vi "Husky Loop.vi"() -> ()   [LabVIEW 2012]
uses:
  clearpath_interface.lvlib
  <vilib>/Platform/TimedLoop/XDataNode/XDataNode.xnode
  <vilib>/Platform/TimedLoop/XDataNode/nitl_modes.ctl
  <vilib>/Platform/TimedLoop/XDataNode/XDNodeRunTimeDep.lvlib
  <vilib>/Platform/TimedLoop/XDataNode/wakeup.ctl
  <vilib>/Platform/TimedLoop/XDataNode/timing_clust.ctl
panel:
  out "Flags":u8 format="%b"
  out "Capacity":i16
  out "Charge":dbl(slide) scale=0.0..100.0
  in  "Debug":bool
  in  "VISA resource name":refnum<visa-resource-name>
  out "Telemetry":T1={"Voltage"={0.0, 0.0, 0.0}, "Encoder Speed"={0, 0}, "Temps"={"IC Temp (C)"=0, "Ch1 Temp (C)"=0, "Ch2 Temp (C)"=0}, "Current"={0.0, 0.0, 0.0, 4.6238981750249924e+36}} {"Current" scale=0.0..16.0; "Temps"."IC Temp (C)" scale=0.0..150.0; "Temps"."Ch1 Temp (C)" scale=0.0..150.0; "Temps"."Ch2 Temp (C)" scale=0.0..150.0; "Encoder Speed" scale=-100.0..100.0; "Voltage" scale=8.0..14.0}
  in  "End Loop":bool
  in  "stop?":bool
  in  "Reset":bool
  in  "Max Accel":dbl
  in  "Set Max Accel":bool
  in  "Max Speed":dbl
  in  "Set Max Speed":bool
  in  "Set Velocity":bool
  in  "Translational Speed":dbl
  in  "Rotational Speed":dbl
  in  "Set Brake":bool
  in  "Continuous Vel":bool
  in  "Right Output":dbl
  in  "Left Output":dbl
  in  "Continuous Output":bool
  in  "Set Output":bool
  in  "P":dbl
  in  "I":dbl
  in  "D":dbl
  in  "FF":dbl
  in  "Stic":dbl
  in  "Int Lim":dbl
  in  "Set Controls":bool
  in  "Right Speed":dbl
  in  "Left Speed":dbl
  in  "Left Accel":dbl
  in  "Right Accel":dbl
  in  "Continuous Speeds":bool
  in  "Set Speeds":bool
  in  "Remote E-Stop":bool
  in  "Set Safety":bool
  in  "New Chassis Time (ms)":u32
  in  "Set Time":bool
  in  "New Chassis Name":string
  in  "Set Name":bool
  in  "FreqRawEncoder":u8
  in  "Update Raw Encoders":bool
  in  "Update Encoder":bool
  in  "FreqEncoder":u8
  in  "FreqPlatformRot":u8
  in  "Update Platform Rotation":bool
  in  "FreqMaxAccel":u8
  in  "Update Max Accel":bool
  in  "FreqMaxSpeed":u8
  in  "Update Max Speed":bool
  in  "FreqDifferentialOutput":u8
  in  "Update Differential Output":bool
  in  "FreqDifferentialControl":u8
  in  "Update Differential Control":bool
  in  "FreqDifferentialSpeed":u8
  in  "Update Differential Speed":bool
  in  "FreqSafetyStatus":u8
  in  "Update Safety Status":bool
  in  "FreqPowerSystem":u8
  in  "Update Power System":bool
  in  "FreqSystemStatus":u8
  in  "Update System Status":bool
  in  "FreqFirmwareInfo":u8
  in  "Update Firmware Info":bool
  in  "FreqPlatformName":u8
  in  "Update Platform Name":bool
  in  "FreqPlatformInfo":u8
  in  "Update Platform Info":bool
  # "Communication Status"
  # "Set Velocity"
  # "Set Differential Speeds"
  # "Set Chassis Name/Time"
  # "Set Differential Controls"
  # "Set Differential Output"
  # "Set Max Speed/Accel"
  # "Set Safety System"
  # "Reset Processor"
  # "Control Test Panel\nClearpath Control Protocol cRIO Test Interface v1.0\nClearpath Robotics Inc., (c) 2010"
  # "Subscriptions"
  # "Platform Info (0x8001)"
  # "Differential Control (0x8201)"
  # "Platform Name (0x8002)"
  # "Differential Output (0x8202)"
  # "Firmware Info (0x8003)"
  # "Max Speed (0x8210)"
  # "System Status (0x8004)"
  # "Max Accel (0x8211)"
  # "Power System (0x8005)"
  # "Platform Rotation (0x8601)"
  # "Safety System Status (0x8010)"
  # "Encoders (0x8800)"
  # "Differential Speed (0x8200)"
  # "Raw Encoders (0x8801)"
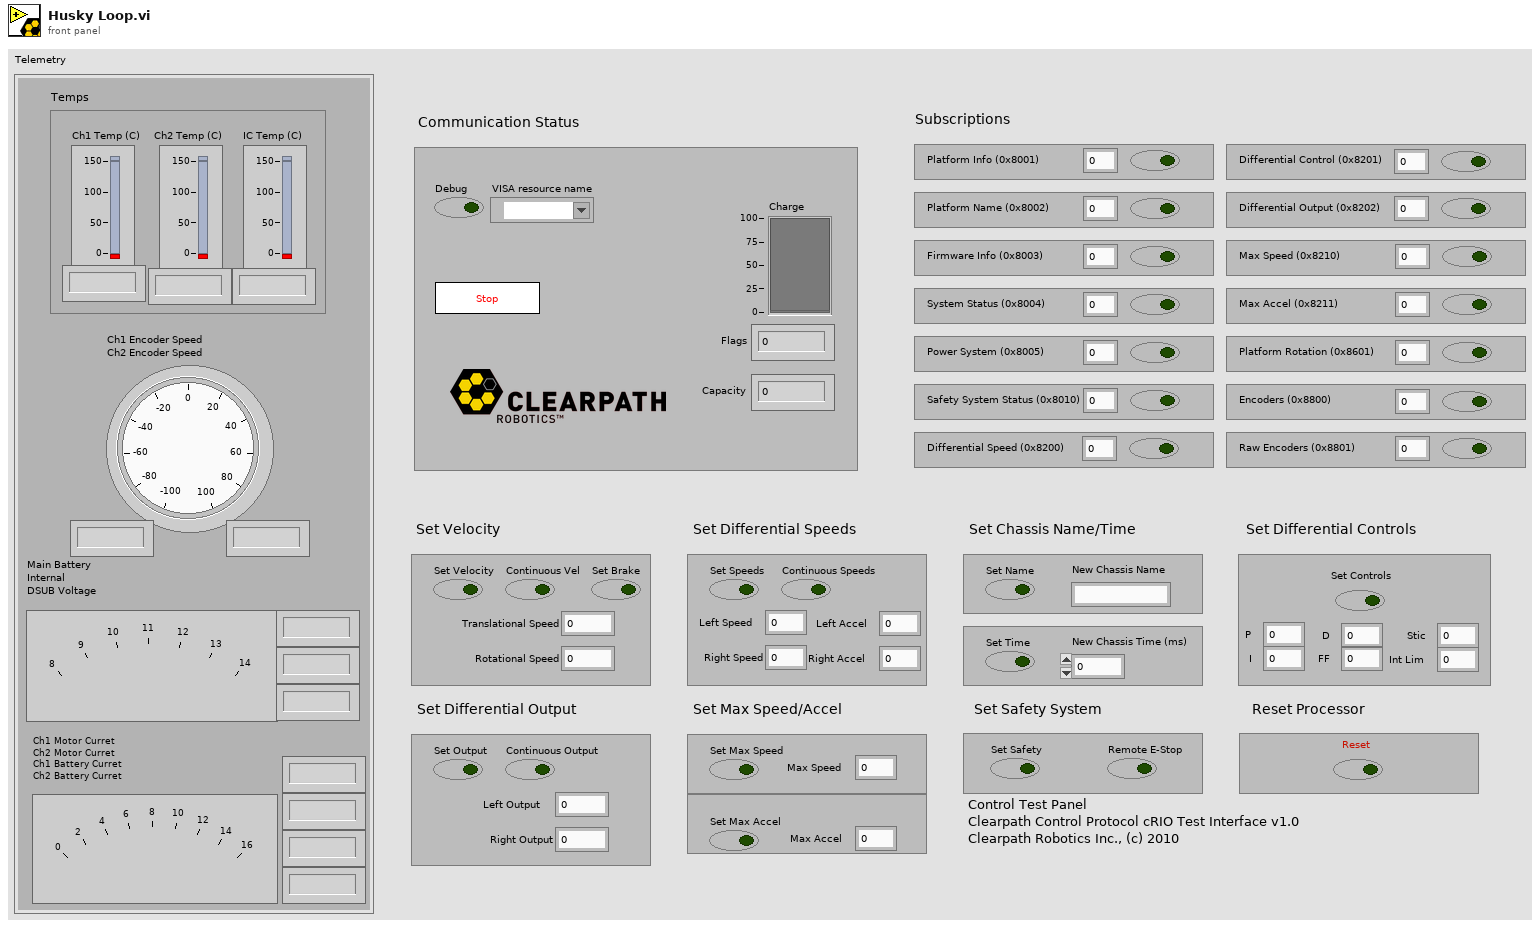
[diagram p1: front panel]
types:
  T1 = cluster{"Voltage":cluster{sgl, sgl, sgl}, "Encoder Speed":cluster{i32, i32}, "Temps":cluster{"IC Temp (C)":i32, "Ch1 Temp (C)":i32, "Ch2 Temp (C)":i32}, "Current":cluster{dbl, dbl, dbl, dbl}}
  T2 = cluster{"Xmit Queue":refnum<queue>, "Data Queue":refnum<queue>, "VISA resource name out":refnum<visa-resource-name>, "error out":errorcluster, "Message Data Cluster":cluster{"\nChar Idx":u8, "Num. Char Rem":u8, "Write Index":u8, "Read Index":u8, "Message Data Buffer":u8[][]}}
  T3 = typedef "XDNodeRunTimeDep.lvlib/timing_clust.ctl" = cluster{"Expected End [f-1]":u64, "Actual End [f-1]":u64, "Finished Late? [f-1]":bool, "Expected End [i-1]":u64, "Actual End [i-1]":u64, "Finished Late? [i-1]":bool, "Expected Start [i]":u64, "Actual Start [i]":u64, "Expected Start [f]":u64, "Actual Start [f]":u64, "Source Name":string, "Structure Name":string, "Period":i64, "Deadline":i64, "Offset":i64, "Start":i64, "Priority":i32, "Timeout":i32, "Mode":T4, "Wakeup Reason":T5, "Error":errorcluster, "Source Type":string, "Secondary Source Type":string, "Global End Time":u64, "Global Start Time":u64, "Frame Duration":u64, "Iteration Duration":u64, "Assigned CPU":i32, "I/O Scan Engine Mode":u32}
  T4 = typedef "XDNodeRunTimeDep.lvlib/nitl_modes.ctl" = enum32{"No Change", "Process missed periods, maintain original phase", "Discard missed periods, maintain original phase", "Process missed periods, ignore original phase", "Discard missed periods, ignore original phase"}
  T5 = typedef "XDNodeRunTimeDep.lvlib/wakeup.ctl" = enum32{"Normal", "Aborted", "Asynchronous wakeup", "Timing source error", "Timed loop error", "Timeout"}
  T6 = cluster{"P":dbl, "I":dbl, "D":dbl, "FF":dbl, "Stic":dbl, "Int Lim":dbl}
  T7 = cluster{"r_p":dbl, "r_i":dbl, "r_d":dbl, "r_ffwd":dbl, "r_stic":dbl, "r_int_lim":dbl}
  T8 = cluster{"l_p":dbl, "l_i":dbl, "l_d":dbl, "l_ffwd":dbl, "l_stic":dbl, "l_int_lim":dbl}
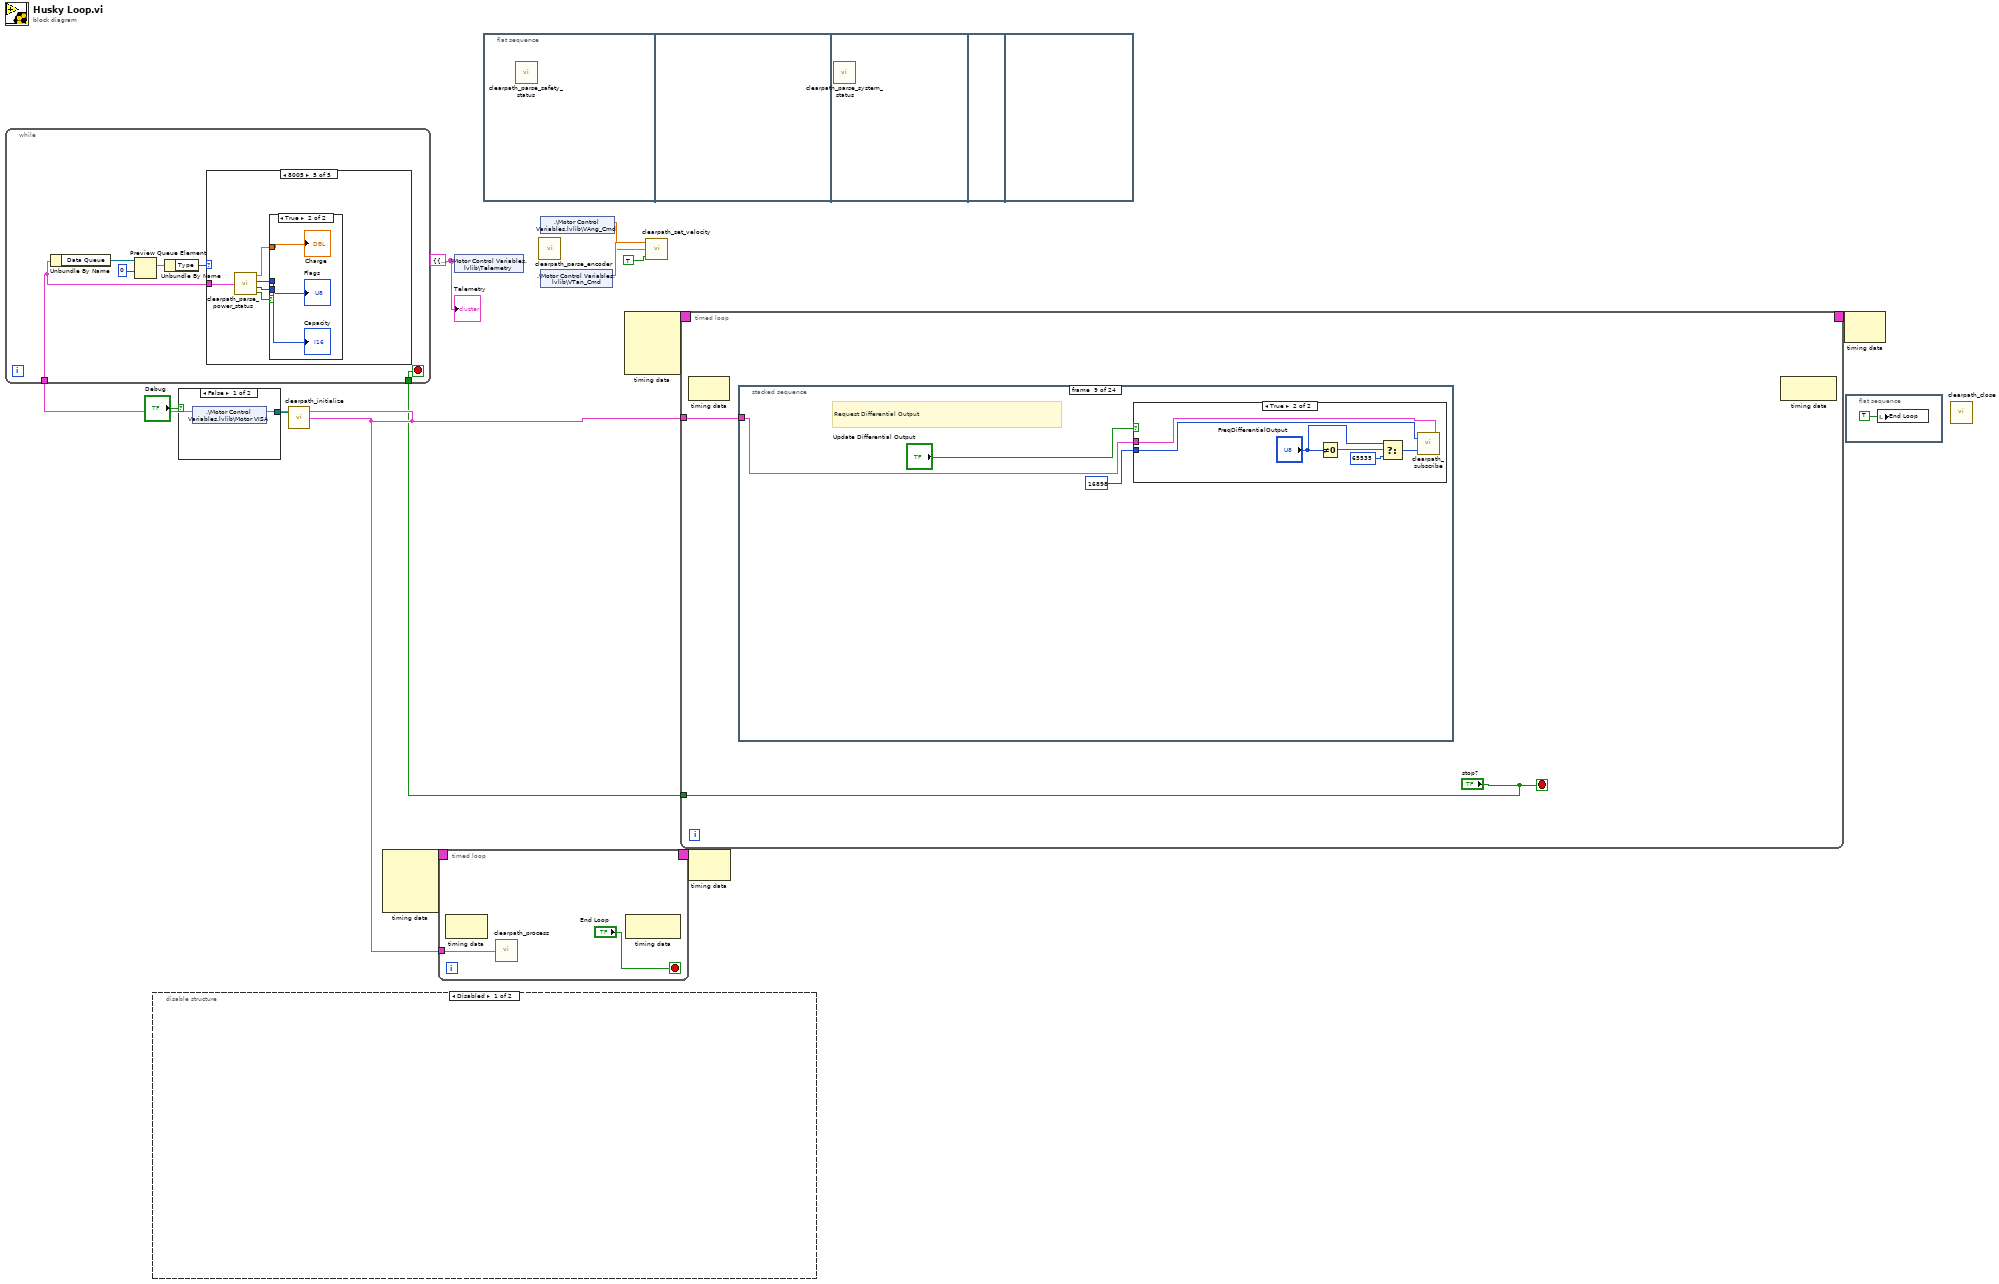
[diagram p0: block diagram]
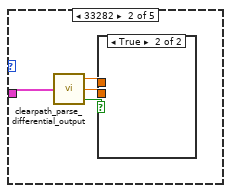
[diagram p3: hidden frame]
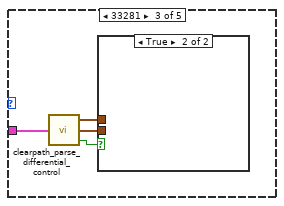
[diagram p5: hidden frame]
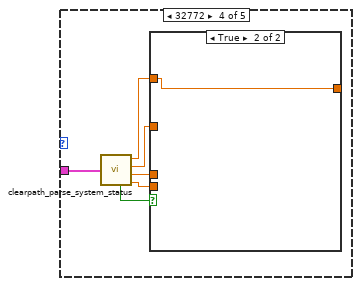
[diagram p7: hidden frame]
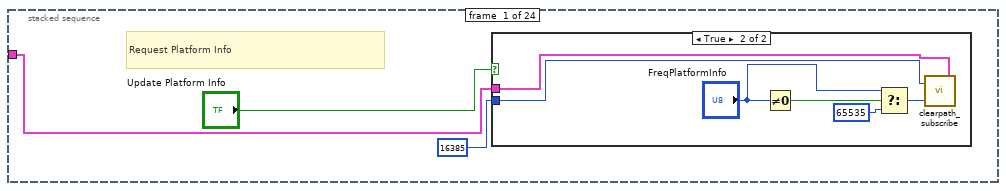
[diagram p10: hidden frame]
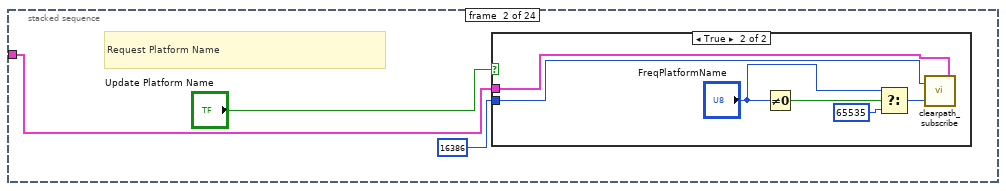
[diagram p12: hidden frame]
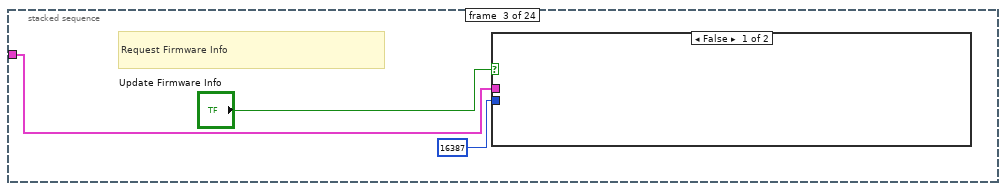
[diagram p14: hidden frame]
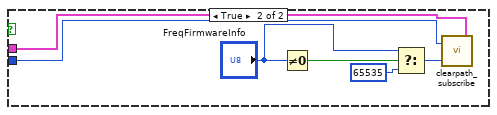
[diagram p15: hidden frame]
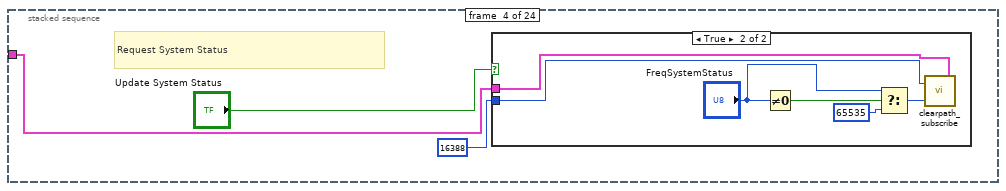
[diagram p16: hidden frame]
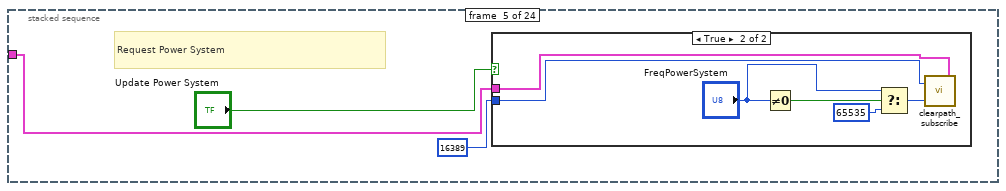
[diagram p18: hidden frame]
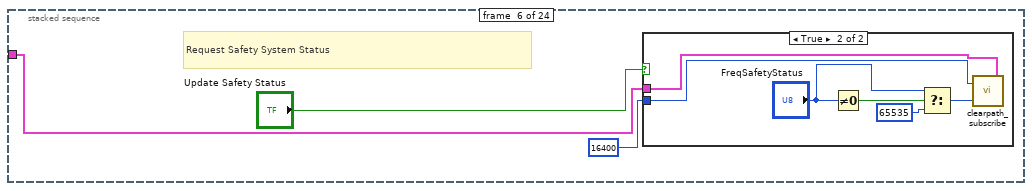
[diagram p20: hidden frame]
diagram:
  w2 = T1 {"Voltage"={0.0, 0.0, 0.0}, "Encoder Speed"={0, 0}, "Temps"={"IC Temp (C)"=0, "Ch1 Temp (C)"=0, "Ch2 Temp (C)"=0}, "Current"={0.0, 0.0, 0.0, 0.0}} ("Telemetry")
  n1 = disable-structure shown="Disabled" {
    frame Disabled {
    }
    frame Enabled {
    }
  }
  n2 = case shown="False" "Debug" {
    tunnel: [w13 "VISA resource name"] -> w11
    frame False {
      n3 = shared-variable ".\\Motor Control Variables.lvlib\\Motor VISA"() -> (w13:refnum<visa-resource-name>)  [unwired: 1 in, 1 out]
    }
    frame True {
    }
  }
  n4 = call "clearpath_initialize.vi"("VISA resource name"=w11) -> ("ClearpathComm"=w3:T2)  [unwired: 1 in]
  n5 = node-c288() -> (w10:T3)  [unwired: 4 in]
  n6 = timed-loop {
    tunnel: w3 -> [w16]
    timing: w10 -> [_]
    timing-out: [_] -> w9
    stop <- "End Loop" stop-if-true
    n7 = node-c288() -> ()  [unwired: 1 in, 1 out]
    n8 = call "clearpath_process.vi"("ClearpathComm"=w16) -> ()
    n9 = node-c288() -> ()  [unwired: 1 in, 1 out]
  }
  n10 = shared-variable ".\\Motor Control Variables.lvlib\\Telemetry"(w2) -> ()  [unwired: 1 in, 1 out]
  n11 = flat-sequence {
    frame #0 {
      n12 = call "clearpath_parse_safety_status.vi"() -> ()  [unwired: 1 in, 2 out]
    }
    frame #1 {
    }
    frame #2 {
      n13 = call "clearpath_parse_system_status.vi"() -> ()  [unwired: 1 in, 6 out]
    }
    frame #3 {
    }
    frame #4 {
    }
  }
  n14 = call "clearpath_parse_encoder.vi"() -> ()  [unwired: 1 in, 5 out]
  n15 = shared-variable ".\\Motor Control Variables.lvlib\\VAng_Cmd"() -> (w5:dbl)  [unwired: 1 in, 1 out]
  n16 = shared-variable ".\\Motor Control Variables.lvlib\\VTan_Cmd"() -> (w6:dbl)  [unwired: 1 in, 1 out]
  n17 = node-c288() -> (w8:T3)  [unwired: 4 in]
  n18 = call "clearpath_set_velocity.vi"("Zero Speeds"=TRUE, "Rotational Speed"=w5, "Translational Speed"=w6) -> ()  [unwired: 1 in]
  n19 = timed-loop {
    tunnel: w3 -> [w20]
    timing: w8 -> [_]
    timing-out: [_] -> w7
    tunnel: ["stop?"] -> w1
    stop <- "stop?" stop-if-true
    n20 = node-c288() -> ()  [unwired: 1 in, 1 out]
    n21 = stacked-sequence {
      tunnel: w20 -> [w24 w34 w42 w51 w60 w69 w78 w87 w96 w105 w114 w124 w133 w142 w150 w154 w158 w163 w170 w181 w187 w194 w198 w202]
      frame #0 {
        # "Request Platform Info"
        n22 = case shown="True" "Update Platform Info" {
          tunnel: w24 -> [_ w26]
          tunnel: 16385 -> [_ w31]
          frame False {
          }
          frame True {
            n23 = Not Equal To 0?(x="FreqPlatformInfo") -> (x != 0?=w29:bool)
            n24 = Select(t="FreqPlatformInfo", s=w29, f=u16 65535) -> (s? t:f=w28:u16)
            n25 = call "clearpath_subscribe.vi"("ClearpathComm"=w26, "Frequency"=w28, "Message Type"=w31) -> ()
          }
        }
      }
      frame #1 {
        # "Request Platform Name"
        n26 = case shown="True" "Update Platform Name" {
          tunnel: w34 -> [_ w35]
          tunnel: 16386 -> [_ w40]
          frame False {
          }
          frame True {
            n27 = Not Equal To 0?(x="FreqPlatformName") -> (x != 0?=w38:bool)
            n28 = Select(t="FreqPlatformName", s=w38, f=u16 65535) -> (s? t:f=w37:u16)
            n29 = call "clearpath_subscribe.vi"("ClearpathComm"=w35, "Frequency"=w37, "Message Type"=w40) -> ()
          }
        }
      }
      frame #2 {
        # "Request Firmware Info"
        n30 = case shown="False" "Update Firmware Info" {
          tunnel: w42 -> [_ w44]
          tunnel: 16387 -> [_ w49]
          frame False {
          }
          frame True {
            n31 = Not Equal To 0?(x="FreqFirmwareInfo") -> (x != 0?=w47:bool)
            n32 = Select(t="FreqFirmwareInfo", s=w47, f=u16 65535) -> (s? t:f=w46:u16)
            n33 = call "clearpath_subscribe.vi"("ClearpathComm"=w44, "Frequency"=w46, "Message Type"=w49) -> ()
          }
        }
      }
      frame #3 {
        # "Request System Status"
        n34 = case shown="True" "Update System Status" {
          tunnel: w51 -> [_ w53]
          tunnel: 16388 -> [_ w58]
          frame False {
          }
          frame True {
            n35 = Not Equal To 0?(x="FreqSystemStatus") -> (x != 0?=w56:bool)
            n36 = Select(t="FreqSystemStatus", s=w56, f=u16 65535) -> (s? t:f=w55:u16)
            n37 = call "clearpath_subscribe.vi"("ClearpathComm"=w53, "Frequency"=w55, "Message Type"=w58) -> ()
          }
        }
      }
      frame #4 {
        # "Request Power System"
        n38 = case shown="True" "Update Power System" {
          tunnel: w60 -> [_ w62]
          tunnel: 16389 -> [_ w67]
          frame False {
          }
          frame True {
            n39 = Not Equal To 0?(x="FreqPowerSystem") -> (x != 0?=w65:bool)
            n40 = Select(t="FreqPowerSystem", s=w65, f=u16 65535) -> (s? t:f=w64:u16)
            n41 = call "clearpath_subscribe.vi"("ClearpathComm"=w62, "Frequency"=w64, "Message Type"=w67) -> ()
          }
        }
      }
      frame #5 {
        # "Request Safety System Status"
        n42 = case shown="True" "Update Safety Status" {
          tunnel: w69 -> [_ w71]
          tunnel: 16400 -> [_ w76]
          frame False {
          }
          frame True {
            n43 = Not Equal To 0?(x="FreqSafetyStatus") -> (x != 0?=w74:bool)
            n44 = Select(t="FreqSafetyStatus", s=w74, f=u16 65535) -> (s? t:f=w73:u16)
            n45 = call "clearpath_subscribe.vi"("ClearpathComm"=w71, "Frequency"=w73, "Message Type"=w76) -> ()
          }
        }
      }
      frame #6 {
        # "Request Differential Speed"
        n46 = case shown="True" "Update Differential Speed" {
          tunnel: w78 -> [_ w80]
          tunnel: 16896 -> [_ w85]
          frame False {
          }
          frame True {
            n47 = Not Equal To 0?(x="FreqDifferentialSpeed") -> (x != 0?=w83:bool)
            n48 = Select(t="FreqDifferentialSpeed", s=w83, f=u16 65535) -> (s? t:f=w82:u16)
            n49 = call "clearpath_subscribe.vi"("ClearpathComm"=w80, "Frequency"=w82, "Message Type"=w85) -> ()
          }
        }
      }
      frame #7 {
        # "Request Differential Control"
        n50 = case shown="True" "Update Differential Control" {
          tunnel: w87 -> [_ w89]
          tunnel: 16897 -> [_ w94]
          frame False {
          }
          frame True {
            n51 = Not Equal To 0?(x="FreqDifferentialControl") -> (x != 0?=w92:bool)
            n52 = Select(t="FreqDifferentialControl", s=w92, f=u16 65535) -> (s? t:f=w91:u16)
            n53 = call "clearpath_subscribe.vi"("ClearpathComm"=w89, "Frequency"=w91, "Message Type"=w94) -> ()
          }
        }
      }
      frame #8 {
        # "Request Differential Output"
        n54 = case shown="True" "Update Differential Output" {
          tunnel: w96 -> [_ w98]
          tunnel: 16898 -> [_ w103]
          frame False {
          }
          frame True {
            n55 = Not Equal To 0?(x="FreqDifferentialOutput") -> (x != 0?=w101:bool)
            n56 = Select(t="FreqDifferentialOutput", s=w101, f=u16 65535) -> (s? t:f=w100:u16)
            n57 = call "clearpath_subscribe.vi"("ClearpathComm"=w98, "Frequency"=w100, "Message Type"=w103) -> ()
          }
        }
      }
      frame #9 {
        # "Request Max Speed"
        n58 = case shown="False" "Update Max Speed" {
          tunnel: w105 -> [_ w107]
          tunnel: 16912 -> [_ w112]
          frame False {
          }
          frame True {
            n59 = Not Equal To 0?(x="FreqMaxSpeed") -> (x != 0?=w110:bool)
            n60 = Select(t="FreqMaxSpeed", s=w110, f=u16 65535) -> (s? t:f=w109:u16)
            n61 = call "clearpath_subscribe.vi"("ClearpathComm"=w107, "Frequency"=w109, "Message Type"=w112) -> ()
          }
        }
      }
      frame #10 {
        # "Request Max Accel"
        n62 = case shown="False" "Update Max Accel" {
          tunnel: w114 -> [_ w116]
          tunnel: 16913 -> [_ w121]
          frame False {
          }
          frame True {
            n63 = Not Equal To 0?(x="FreqMaxAccel") -> (x != 0?=w119:bool)
            n64 = Select(t="FreqMaxAccel", s=w119, f=u16 65535) -> (s? t:f=w118:u16)
            n65 = call "clearpath_subscribe.vi"("ClearpathComm"=w116, "Frequency"=w118, "Message Type"=w121) -> ()
          }
        }
      }
      frame #11 {
        # "Request Platform Rotation"
        n66 = case shown="False" "Update Platform Rotation" {
          tunnel: w124 -> [_ w125]
          tunnel: 17921 -> [_ w130]
          frame False {
          }
          frame True {
            n67 = Not Equal To 0?(x="FreqPlatformRot") -> (x != 0?=w128:bool)
            n68 = Select(t="FreqPlatformRot", s=w128, f=u16 65535) -> (s? t:f=w127:u16)
            n69 = call "clearpath_subscribe.vi"("ClearpathComm"=w125, "Frequency"=w127, "Message Type"=w130) -> ()
          }
        }
      }
      frame #12 {
        # "Request Encoders"
        n70 = case shown="False" "Update Encoder" {
          tunnel: w133 -> [_ w134]
          tunnel: 18432 -> [_ w139]
          frame False {
          }
          frame True {
            n71 = Not Equal To 0?(x="FreqEncoder") -> (x != 0?=w136:bool)
            n72 = Select(t="FreqEncoder", s=w136, f=u16 65535) -> (s? t:f=w135:u16)
            n73 = call "clearpath_subscribe.vi"("ClearpathComm"=w134, "Frequency"=w135, "Message Type"=w139) -> ()
          }
        }
      }
      frame #13 {
        # "Request Raw Encoders"
        n74 = case shown="False" "Update Raw Encoders" {
          tunnel: w142 -> [_ w143]
          tunnel: 18433 -> [_ w148]
          frame False {
          }
          frame True {
            n75 = Not Equal To 0?(x="FreqRawEncoder") -> (x != 0?=w146:bool)
            n76 = Select(t="FreqRawEncoder", s=w146, f=u16 65535) -> (s? t:f=w145:u16)
            n77 = call "clearpath_subscribe.vi"("ClearpathComm"=w143, "Frequency"=w145, "Message Type"=w148) -> ()
          }
        }
      }
      frame #14 {
        # "Set Platform Name"
        n78 = case shown="True" "Set Name" {
          tunnel: w150 -> [_ w151]
          frame False {
          }
          frame True {
            n79 = call "clearpath_set_platform_name.vi"("ClearpathComm"=w151, "New Name"="New Chassis Name") -> ()
          }
        }
      }
      frame #15 {
        # "Set Platform Time"
        n80 = case shown="True" "Set Time" {
          tunnel: w154 -> [_ w155]
          frame False {
          }
          frame True {
            n81 = call "clearpath_set_platform_time.vi"("ClearpathComm"=w155, "New Time"="New Chassis Time (ms)") -> ()
          }
        }
      }
      frame #16 {
        # "Set Safety System"
        n82 = case shown="True" "Set Safety" {
          tunnel: w158 -> [_ _]
          frame False {
          }
          frame True {
            n83 = call "clearpath_set_safety_system.vi"("Set Stop Flag"="Remote E-Stop") -> ()  [unwired: 1 in]
          }
        }
      }
      frame #17 {
        # "Set Differential Speeds"
        n84 = Or(x="Continuous Speeds", y="Set Speeds") -> (x .or. y?=w161:bool)
        n85 = case shown="True" w161 {
          tunnel: w163 -> [_ w164]
          frame False {
          }
          frame True {
            n86 = call "clearpath_set_differential_speeds.vi"("ClearpathComm"=w164, "Right Accel"="Right Accel", "Left Accel"="Left Accel", "Right Speed"="Right Speed", "Left Speed"="Left Speed") -> ()
          }
        }
      }
      frame #18 {
        # "Set Differential Controls"
        n87 = case shown="False" "Set Controls" {
          tunnel: w170 -> [_ _]
          frame False {
          }
          frame True {
            n88 = Bundle("P"="P", "I"="I", "D"="D", "FF"="FF", "Stic"="Stic", "Int Lim"="Int Lim") -> (w171:T6)  [unwired: 1 in]
            n89 = call "clearpath_set_differential_controls.vi"("Controls Cluster"=w171) -> ()  [unwired: 1 in]
          }
        }
      }
      frame #19 {
        # "Set Differential Output"
        n90 = Or(x="Continuous Output", y="Set Output") -> (x .or. y?=w179:bool)
        n91 = case shown="True" w179 {
          tunnel: w181 -> [_ w182]
          frame False {
          }
          frame True {
            n92 = call "clearpath_set_differential_output.vi"("ClearpathComm"=w182, "Right Output"="Right Output", "Left Output"="Left Output") -> ()
          }
        }
      }
      frame #20 {
        # "Set Velocity"
        n93 = Or(x="Continuous Vel", y="Set Velocity") -> (x .or. y?=w186:bool)
        n94 = case shown="True" w186 {
          tunnel: w187 -> [_ w189]
          frame False {
          }
          frame True {
            n95 = call "clearpath_set_velocity.vi"("ClearpathComm"=w189, "Zero Speeds"="Set Brake", "Rotational Speed"="Rotational Speed", "Translational Speed"="Translational Speed") -> ()
          }
        }
      }
      frame #21 {
        # "Set Max Speed"
        n96 = case shown="True" "Set Max Speed" {
          tunnel: w194 -> [_ w195]
          frame False {
          }
          frame True {
            n97 = call "clearpath_set_max_speed.vi"("ClearpathComm"=w195, "Max Speed"="Max Speed") -> ()
          }
        }
      }
      frame #22 {
        # "Set Max Accel"
        n98 = case shown="True" "Set Max Accel" {
          tunnel: w198 -> [_ w199]
          frame False {
          }
          frame True {
            n99 = call "clearpath_set_max_accel.vi"("ClearpathComm"=w199, "Max Accel"="Max Accel") -> ()
          }
        }
      }
      frame #23 {
        # "Reset Processor"
        n100 = case shown="True" "Reset" {
          tunnel: w202 -> [_ _]
          frame False {
          }
          frame True {
          }
        }
      }
    }
    n101 = node-c288() -> ()  [unwired: 1 in, 1 out]
  }
  n102 = while {
    tunnel: w3 -> [w204]
    tunnel: w1 -> [w203]
    stop <- w203 stop-if-true
    n103 = Unbundle By Name(w204) -> ("Data Queue"=w205:refnum<queue>)
    n104 = Preview Queue Element(queue=w205, timeout in ms (-1)=0) -> (element=w207:cluster{u8[], "Length":i32, "Type":i32})  [unwired: 1 in, 3 out]
    n105 = Unbundle By Name(w207) -> ("Type"=w208:i32)
    n106 = case shown="8005" w208 {
      tunnel: w204 -> [_ w212 w216 w222 w225]
      frame 0, Default {
      }
      frame 33282 {
        n107 = call "clearpath_parse_differential_output.vi"("ClearpathComm"=w212) -> ("Data Valid?"=w209:bool, "Right Output"=w210:dbl, "Left Output"=w211:dbl)
        n108 = case shown="True" w209 {
          tunnel: w211 -> [_ _]
          tunnel: w210 -> [_ _]
          frame False {
          }
          frame True {
          }
        }
      }
      frame 33281 {
        n109 = call "clearpath_parse_differential_control.vi"("ClearpathComm"=w216) -> ("Data Valid?"=w215:bool, "Right Controls"=w214:T7, "Left Controls"=w213:T8)
        n110 = case shown="True" w215 {
          tunnel: w214 -> [_ _]
          tunnel: w213 -> [_ _]
          frame False {
          }
          frame True {
          }
        }
      }
      frame 32772 {
        n111 = call "clearpath_parse_system_status.vi"("ClearpathComm"=w222) -> ("Data Valid?"=w221:bool, "Right Motor Current"=w218:dbl, "Left Motor Current"=w217:dbl, "Controls Current"=w219:dbl, "Battery Voltage"=w220:dbl)  [unwired: 1 out]
        n112 = case shown="True" w221 {
          tunnel: w220 -> [_ w223]
          tunnel: w219 -> [_ _]
          tunnel: w218 -> [_ _]
          tunnel: w217 -> [_ _]
          tunnel: [_ w223] -> _
          frame False {
          }
          frame True {
          }
        }
      }
      frame 32773 {
        n113 = call "clearpath_parse_power_status.vi"("ClearpathComm"=w225) -> ("Data Valid?"=w224:bool, "Capacity"=w226:i16, "Flags"=w227:u8, "Charge"=w228:dbl)
        n114 = case shown="True" w224 {
          tunnel: w228 -> [_ w231]
          tunnel: w227 -> [_ w229]
          tunnel: w226 -> [_ w230]
          frame False {
          }
          frame True {
            "Flags" <- w229
            "Capacity" <- w230
            "Charge" <- w231
          }
        }
      }
    }
  }
  n115 = node-c288(w9) -> ()  [unwired: 1 out]
  n116 = node-c288(w7) -> ()  [unwired: 1 out]
  n117 = flat-sequence {
    frame #0 {
      n118 = local write "End Loop"(TRUE ("End Loop")) -> ()
    }
  }
  n119 = call "clearpath_close.vi"() -> ()  [unwired: 1 in]
  "Telemetry" <- w2
